vi "test Controller.vi"() -> ()   [LabVIEW 2017, in "SampleRotator.lvlib"]
uses:
  SampleRotator.lvlib
  ctl/Rotator controller info.ctl
  ctl/Motion Properties.ctl
  ctl/Positoin to set.ctl
  ctl/Axis status.ctl
  Messenger service/Data types/MSG to TOP.ctl
  Messenger service/Data types/Module name.ctl
  ctl/Rotator commands.ctl
  Messenger service/MessengerLib.lvlib
panel:
  out "Position":T1
  out "parameters":T2={"Amplitude [V]"=5.0, "DC voltage [V]"=0.0, "Precision [m°]"=100.0, "Frequency [Hz]"=1000.0} {"Amplitude [V]" min=0.0 max=60.0; "DC voltage [V]" min=0.0 max=60.0; "Precision [m°]" min=1.0 max=1000.0; "Frequency [Hz]" min=0.1 max=5000.0}
  out "Last response":T3
  in  "Stop":bool
  out "Axis status":T5
  in  "Set parameters":bool
  in  "Set position":T1
  in  "Motion properties":T2={"Amplitude [V]"=5.0, "DC voltage [V]"=0.0, "Precision [m°]"=100.0, "Frequency [Hz]"=1000.0} {"Amplitude [V]" min=0.0 max=60.0; "DC voltage [V]" min=0.0 max=60.0; "Precision [m°]" min=1.0 max=1000.0; "Frequency [Hz]" min=0.1 max=5000.0}
  out "Actuator info":T6 {"DeviceType" items=["ANC350res", "ANC350num", "ANC350fps", "No device / invalid"]; "ID" format="%x"}
  in  "Connect":bool
  in  "Disconnect":bool
  in  "set position":bool
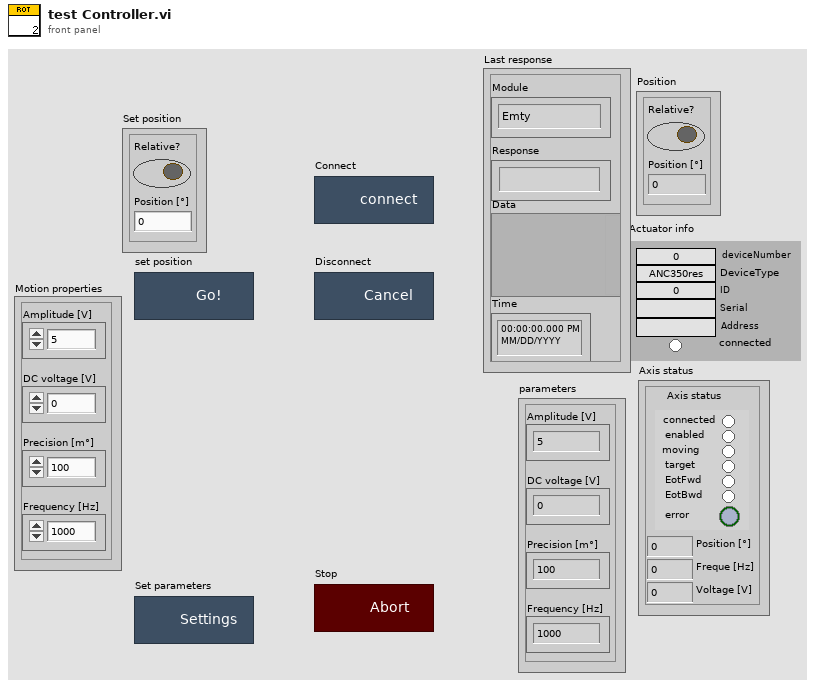
[diagram p1: front panel]
types:
  T1 = typedef "Positoin to set.ctl" = cluster{"Relative?":bool, "Position [°]":dbl}
  T2 = typedef "Motion Properties.ctl" = cluster{"Amplitude [V]":dbl, "DC voltage [V]":dbl, "Precision [m°]":dbl, "Frequency [Hz]":dbl}
  T3 = typedef "MessengerLib.lvlib/MSG to TOP.ctl" = cluster{"Module":T4, "Response":string, "Data":variant, "Time":timestamp}
  T4 = typedef "MessengerLib.lvlib/Module name.ctl" = enum16{"Emty", "Magnet", "VTI", "Excitation", "Servo", "Acquisition", "Rotator", "Digitizer"}
  T5 = typedef "SampleRotator.lvlib/Axis status.ctl" = cluster{"Axis status":cluster{"connected":bool, "enabled":bool, "moving":bool, "target":bool, "EotFwd":bool, "EotBwd":bool, "error":bool}, "Position [°]":dbl, "Freque [Hz]":dbl, "Voltage [V]":dbl}
  T6 = typedef "SampleRotator.lvlib/Rotator controller info.ctl" = cluster{"deviceNumber":i32, "DeviceType":i32, "ID":u32, "Serial":string, "Address":string, "connected":bool}
  T7 = typedef "MessengerLib.lvlib/Messenger referencies.ctl" = cluster{"Magnet":refnum<queue>, "VTI":refnum<queue>, "Excitation":refnum<queue>, "ACQ":refnum<queue>, "Servo":refnum<queue>, "Rotator":refnum<queue>, "Top":refnum<queue>}
  T8 = typedef "SampleRotator.lvlib/Rotator commands.ctl" = enum16{"Ignore", "Initialize", "Update", "Set parameters", "Stop movement", "Set position", "End"}
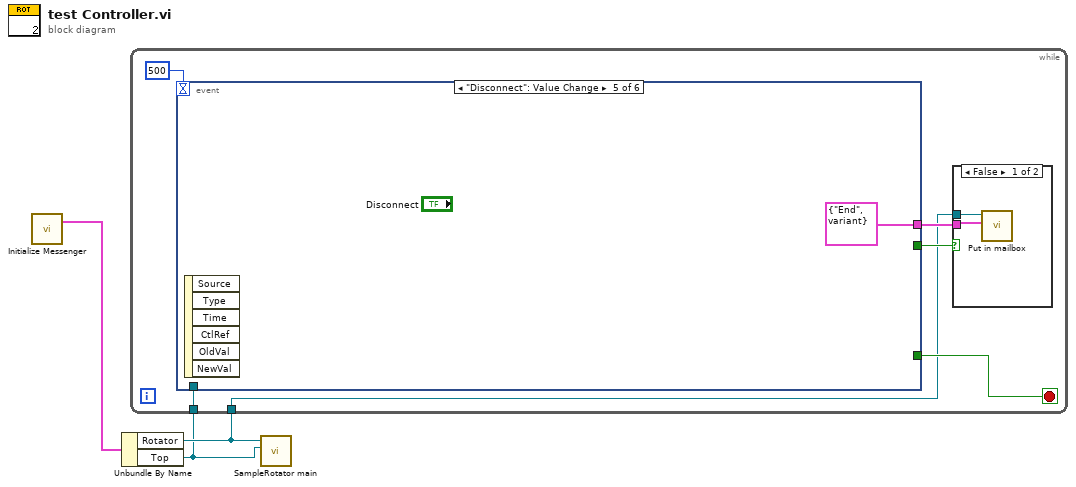
[diagram p0: block diagram]
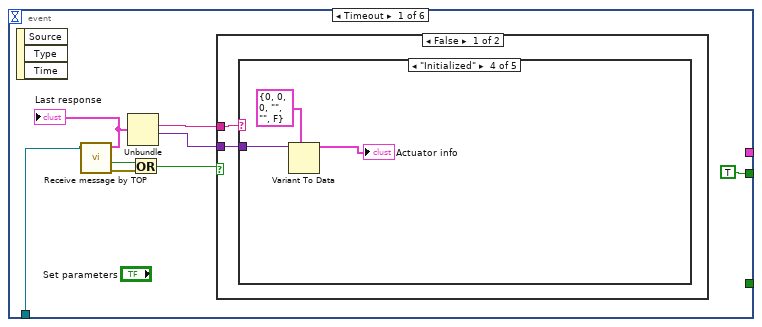
[diagram p3: hidden frame]
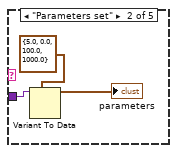
[diagram p5: hidden frame]
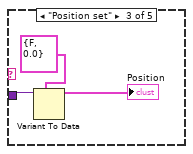
[diagram p6: hidden frame]
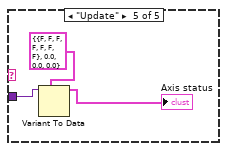
[diagram p7: hidden frame]
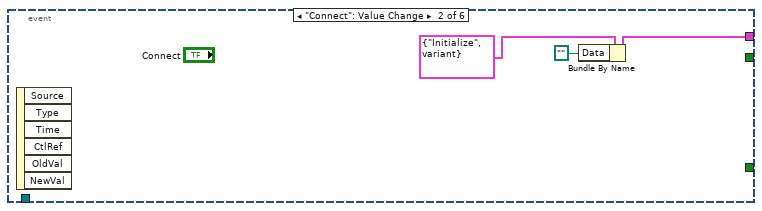
[diagram p9: hidden frame]
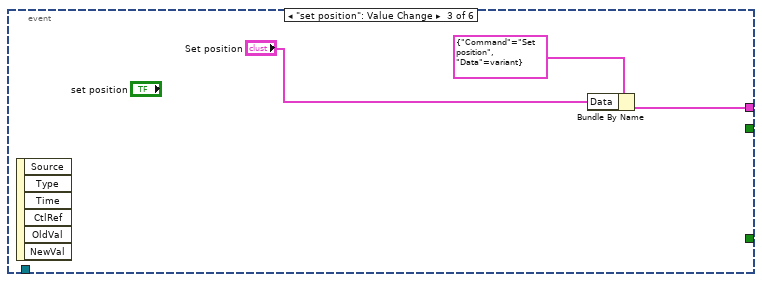
[diagram p10: hidden frame]
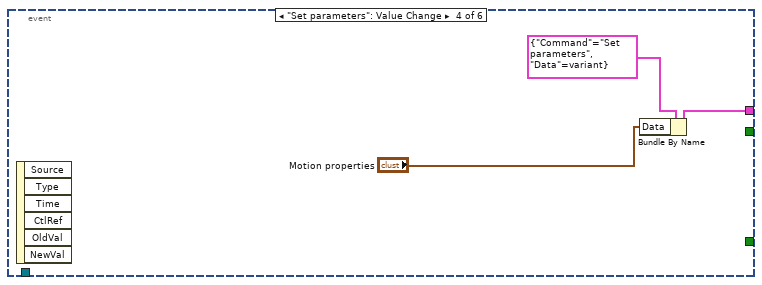
[diagram p11: hidden frame]
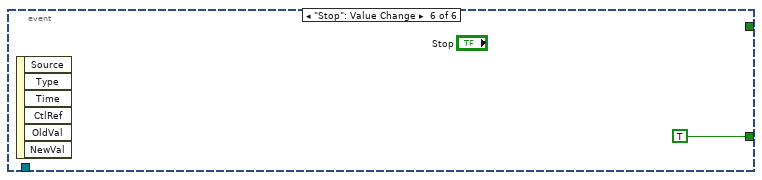
[diagram p12: hidden frame]
diagram:
  n1 = call "Initialize Messenger.vi"() -> ("Referencies out"=w3:T7)  [unwired: 2 in, 1 out]
  n2 = Unbundle By Name(w3) -> ("Rotator"=w2:refnum<queue>, "Top"=w1:refnum<queue>)
  n3 = while {
    tunnel: w2 -> [w5]
    tunnel: w1 -> [w4]
    stop <- w7 stop-if-true
    n4 = event shown="[4] \"Disconnect\": Value Change" {
      selector: _ -> [_ _ _ _ _ _]
      dyn-events: _ -> [_ _ _ _ _ _]
      timeout: 500 -> [_ _ _ _ _ _]
      tunnel: [TRUE _ _ _ _ _] -> w9
      tunnel: [_ w35 w38 w41 cluster{"Command":T8, "Data":variant} {"Command"=enum."End", "Data"=variant} ("MSG to rotator") _] -> w8
      tunnel: [_ _ _ _ _ TRUE] -> w7
      tunnel: w4 -> [w13 _ _ _ _ _]
      event Timeout {
        n5 = event-data() -> ()  [unwired: 1 in, 3 out]
        n6 = call "Receive message by TOP.vi"("Mailbox in"=w13) -> ("error out"=w16:errorcluster, "timed out?"=w15:bool, "MSG packet"=w19:T3)  [unwired: 7 in, 1 out]
        "Last response" <- w19
        n7 = Unbundle(w19) -> ("Response"=w18:string, "Data"=w12:variant)  [unwired: 2 out]
        n8 = Or(x=w15, y=w16) -> (x .or. y?=w17:bool)
        n9 = case shown="False" w17 {
          tunnel: w18 -> [w21 _]
          tunnel: w12 -> [w20 _]
          frame False {
            n10 = case shown="\"Initialized\"" w21 {
              tunnel: w20 -> [_ w24 w27 w30 w33]
              frame "Ignored", Default {
              }
              frame "Parameters set" {
                n11 = Variant To Data(type=T2 {"Amplitude [V]"=5.0, "DC voltage [V]"=0.0, "Precision [m°]"=100.0, "Frequency [Hz]"=1000.0} ("Motion properties"), Variant=w24) -> (data=→"parameters":T2)  [unwired: 1 in, 1 out]
              }
              frame "Position set" {
                n12 = Variant To Data(type=T1 {"Relative?"=FALSE, "Position [°]"=0.0} ("Set position"), Variant=w27) -> (data=→"Position":T1)  [unwired: 1 in, 1 out]
              }
              frame "Initialized" {
                n13 = Variant To Data(type=T6 {"deviceNumber"=0, "DeviceType"=0, "ID"=0, "Serial"="", "Address"="", "connected"=FALSE} ("Actuator info"), Variant=w30) -> (data=→"Actuator info":T6)  [unwired: 1 in, 1 out]
              }
              frame "Update" {
                n14 = Variant To Data(type=T5 {"Axis status"={"connected"=FALSE, "enabled"=FALSE, "moving"=FALSE, "target"=FALSE, "EotFwd"=FALSE, "EotBwd"=FALSE, "error"=FALSE}, "Position [°]"=0.0, "Freque [Hz]"=0.0, "Voltage [V]"=0.0} ("Axis status 2"), Variant=w33) -> (data=→"Axis status":T5)  [unwired: 1 in, 1 out]
              }
            }
          }
          frame True {
          }
        }
      }
      event "Connect": Value Change {
        n15 = event-data() -> ()  [unwired: 1 in, 6 out]
        n16 = Bundle By Name(cluster=cluster{"Command":T8, "Data":variant} {"Command"=enum."Initialize", "Data"=variant} ("MSG to rotator"), "Data"=path "") -> (w35:cluster{"Command":T8, "Data":variant})
      }
      event "set position": Value Change {
        n17 = event-data() -> ()  [unwired: 1 in, 6 out]
        n18 = Bundle By Name(cluster=cluster{"Command":T8, "Data":variant} {"Command"=enum."Set position", "Data"=variant} ("MSG to rotator"), "Data"="Set position") -> (w38:cluster{"Command":T8, "Data":variant})
      }
      event "Set parameters": Value Change {
        n19 = event-data() -> ()  [unwired: 1 in, 6 out]
        n20 = Bundle By Name(cluster=cluster{"Command":T8, "Data":variant} {"Command"=enum."Set parameters", "Data"=variant} ("MSG to rotator"), "Data"="Motion properties") -> (w41:cluster{"Command":T8, "Data":variant})
      }
      event "Disconnect": Value Change {
        n21 = event-data() -> ()  [unwired: 1 in, 6 out]
      }
      event "Stop": Value Change {
        n22 = event-data() -> ()  [unwired: 1 in, 6 out]
      }
    }
    n23 = case shown="False" w9 {
      tunnel: w5 -> [w11 _]
      tunnel: w8 -> [w10 _]
      frame False {
        n24 = call "Put in mailbox.vi"("Message"=w10, "Queue in"=w11) -> ()  [unwired: 7 in, 3 out]
      }
      frame True {
      }
    }
  }
  n25 = call "SampleRotator main.vi"("Top"=w1, "Rotator"=w2) -> ()  [unwired: 8 in, 2 out]
